vi "_unittest Cache.vi"(7 "Action":T2(ring), 8 "error in (no error)":errorcluster, 9 "Passed?":bool, 10 "Test Details":string, 11 "Test Name":string) -> (0 "error out":errorcluster, 3 "Tests":T1(array[cluster]))   [LabVIEW 2019, in "labview_json_tests.lvlib"]
uses:
  labview_json_tests.lvlib
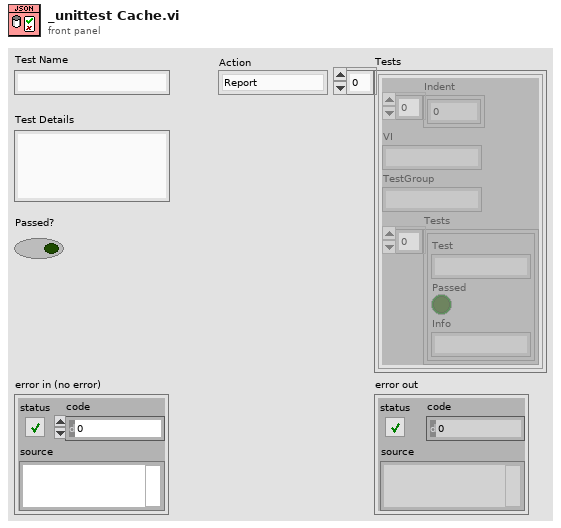
[diagram p1: front panel]
types:
  T1 = cluster{"Indent":i32[], "VI":string, "TestGroup":string, "Tests":cluster{"Test":string, "Passed":bool, "Info":string}[]}[]
  T2 = enum8{"Report", "Add Test Group", "Add Test Case"}
  T3 = cluster{"Indent":i32[], "VI":string, "TestGroup":string, "Tests":cluster{"Test":string, "Passed":bool, "Info":string}[]}
  T4 = cluster{"Test":string, "Passed":bool, "Info":string}
  T5 = cluster{"Test":string, "Passed":bool, "Info":string}[]
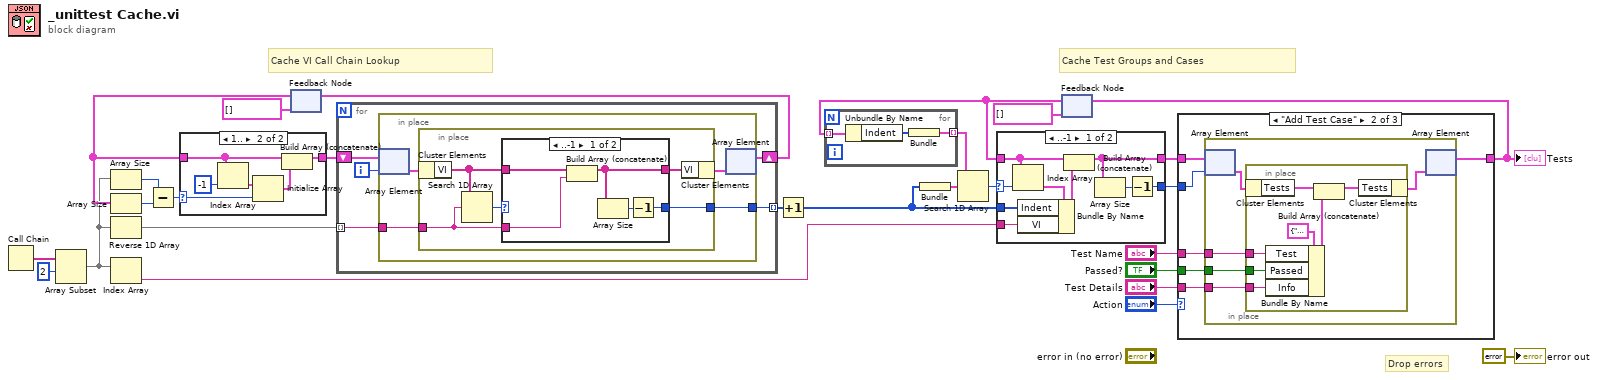
[diagram p0: block diagram]
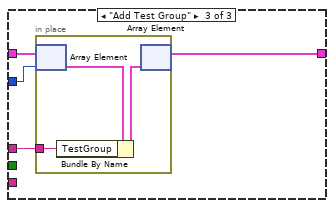
[diagram p4: hidden frame]
diagram:
  # "Drop errors"
  # "Cache Test Groups and Cases"
  # "Cache VI Call Chain Lookup"
  n1 = Call Chain() -> (call chain=w26:string[])
  n2 = Array Subset(array=w26, index=2) -> (w6:string[])  [unwired: 1 in]
  n3 = Array Size(array=w6) -> (size(s)=w14:i32)
  n4 = Reverse 1D Array(array=w6) -> (reversed array=w4:string[])
  n5 = Index Array(array=w6) -> (element=w5:string)  [unwired: 1 in]
  n6 = feedback #1(cluster{"VI":string[]}[] [] ("Array")) -> (w9:cluster{"VI":string[]}[])
  n7 = Array Size(array=w9) -> (size(s)=w13:i32)
  n8 = Subtract(x=w14, y=w13) -> (x-y=w11:i32)
  n9 = case shown="1.." w11 {
    selector: w11 -> [_ w30]
    tunnel: [w28 w34] -> w12
    tunnel: w9 -> [w28 w33]
    frame ..0 {
    }
    frame 1.. {
      n10 = Index Array(array=w33, index=-1) -> (element=w32:cluster{"VI":string[]})
      n11 = Initialize Array(w32, w30) -> (w31:cluster{"VI":string[]}[])
      n12 = Build Array (concatenate)(w33, w31) -> (w34:cluster{"VI":string[]}[])
    }
  }
  n13 = for {
    tunnel: w4 -> [w38] mode=indexing
    shift-right: [w37] -> w8
    shift-left: w12 -> [w39]
    tunnel: [w36] -> w7 mode=indexing
    i -> [w35]
    n14 = in-place {
      in-place-border: w38 -> [w43]
      in-place-border: [w40] -> w36
      n15 = in-place-array #2(w39, w35) -> (w42:cluster{"VI":string[]})
      n16 = in-place {
        in-place-border: w43 -> [w47]
        in-place-border: [w44] -> w40
        n17 = in-place-cluster #3(w42) -> ("VI"=w45:string[])
        n18 = Search 1D Array(1D array=w45, element=w47) -> (index of element=w48:i32)  [unwired: 1 in]
        n19 = case shown="..-1" w48 {
          selector: w48 -> [_ w54]
          tunnel: w47 -> [w52 _]
          tunnel: [w51 w55] -> w46
          tunnel: w45 -> [w53 w55]
          tunnel: [w49 w54] -> w44
          frame ..-1 {
            n20 = Build Array (concatenate)(w53, w52) -> (w51:string[])
            n21 = Array Size(array=w51) -> (size(s)=w50:i32)
            n22 = Decrement(x=w50) -> (x-1=w49:i32)
          }
          frame 0.. {
          }
        }
        n23 = in-place-cluster #3("VI"=w46) -> (w41:cluster{"VI":string[]})
      }
      n24 = in-place-array #2(w41) -> (w37:cluster{"VI":string[]}[])  [unwired: 1 out]
    }
  }
  n25 = feedback-in #1(w8) -> ()
  n26 = Increment(x=w7) -> (x+1=w3:i32[])
  n27 = Bundle(w3) -> (w24:cluster{i32[]})  [unwired: 1 in]
  n28 = feedback #4(T1 [] ("Test 2")) -> (w16:T1)
  n29 = for {
    tunnel: w16 -> [w58] mode=indexing
    tunnel: [w56] -> w15 mode=indexing
    n30 = Unbundle By Name(w58) -> ("Indent"=w57:i32[])
    n31 = Bundle("Indent"=w57) -> (w56:cluster{"Indent":i32[]})  [unwired: 1 in]
  }
  n32 = Search 1D Array(1D array=w15, element=w24) -> (index of element=w23:i32)  [unwired: 1 in]
  n33 = case shown="..-1" w23 {
    selector: w23 -> [w66 w68]
    tunnel: [w63 w69] -> w22
    tunnel: w16 -> [w67 w69]
    tunnel: [w62 w68] -> w21
    tunnel: w5 -> [w60 _]
    tunnel: w3 -> [w59 _]
    frame ..-1 {
      n34 = Index Array(array=w67, index=w66) -> (element=w65:T3)
      n35 = Bundle By Name(cluster=w65, "Indent"=w59, "VI"=w60) -> (w61:T3)
      n36 = Build Array (concatenate)(w67, w61) -> (w63:T1)
      n37 = Array Size(array=w63) -> (size(s)=w64:i32)
      n38 = Decrement(x=w64) -> (x-1=w62:i32)
    }
    frame 0.. {
    }
  }
  n39 = case shown="\"Add Test Case\"" "Action" {
    tunnel: w22 -> [w70 w76 w92]
    tunnel: w21 -> [_ w75 w91]
    tunnel: [w70 w74 w90] -> w20
    tunnel: "Test Name" -> [_ w73 w89]
    tunnel: "Passed?" -> [_ w72 _]
    tunnel: "Test Details" -> [_ w71 _]
    frame "Report" {
    }
    frame "Add Test Case" {
      n40 = in-place {
        in-place-border: w73 -> [w79]
        in-place-border: w72 -> [w78]
        in-place-border: w71 -> [w77]
        n41 = in-place-array #5(w76, w75) -> (w81:T3)
        n42 = in-place {
          in-place-border: w79 -> [w85]
          in-place-border: w78 -> [w84]
          in-place-border: w77 -> [w83]
          n43 = in-place-cluster #6(w81) -> ("Tests"=w87:T5)
          n44 = Bundle By Name(cluster=T4 {"Test"="", "Passed"=FALSE, "Info"=""} ("element"), "Test"=w85, "Passed"=w84, "Info"=w83) -> (w86:T4)
          n45 = Build Array (concatenate)(w87, w86) -> (w88:T5)
          n46 = in-place-cluster #6("Tests"=w88) -> (w80:T3)
        }
        n47 = in-place-array #5(w80) -> (w74:T1)  [unwired: 1 out]
      }
    }
    frame "Add Test Group" {
      n48 = in-place {
        in-place-border: w89 -> [w93]
        n49 = in-place-array #7(w92, w91) -> (w95:T3)
        n50 = Bundle By Name(cluster=w95, "TestGroup"=w93) -> (w94:T3)
        n51 = in-place-array #7(w94) -> (w90:T1)  [unwired: 1 out]
      }
    }
  }
  "Tests" <- w20
  n52 = feedback-in #4(w20) -> ()
  "error out" <- errorcluster {"status"=FALSE, "code"=0, "source"=""} ("error out")
